vi "Vision Processing.vi"(4 "error in (no error)":errorcluster, 7 "Image Size":T1=enum."320x240") -> ()   [LabVIEW 2020]
doc: "This VI runs in parallel to other tasks. It gets images from the camera, processes them for color or shape and uses commands or globals to affect the behavior of other subsystems."
uses:
  <vilib>/Rock Robotics/WPI/Camera/WPI_CameraImageSize.ctl
  <vilib>/Rock Robotics/WPI/Camera/WPI_CameraWhite Balance Values.ctl
  <vilib>/Rock Robotics/WPI/Camera/WPI_CameraExposure Values.ctl
  <vilib>/Rock Robotics/WPI/Camera/WPI_CameraFrameRate.ctl
  Framework/Robot Global Data.vi
  <vilib>/Rock Robotics/Network Tables/NT Read Number.vi
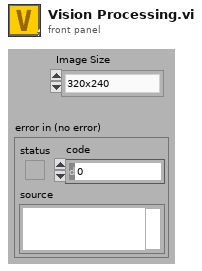
[diagram p1: front panel]
types:
  T1 = typedef "WPI_CameraImageSize.ctl" = enum16{"640x480", "320x240", "160x120", "Custom"}
  T2 = typedef "WPI_CameraFrameRate.ctl" = u32
  T3 = typedef "WPI_CameraExposure Values.ctl" = enum16{"Auto", "Flicker-free 50 Hz", "Flicker-free 60 Hz", "Hold current", "Custom"}
  T4 = typedef "WPI_CameraWhite Balance Values.ctl" = enum16{"Auto", "Fixed indoor", "Fixed outdoor 1", "Fixed outdoor 2", "Fixed fluorescent 1", "Fixed fluorescent 2", "Hold current", "Custom"}
  T5 = typedef "Image Type" = u32
  T6 = typedef "WPI_CameraDevRef.ctl" = cluster{"Camera Address":string, "CameraStatus":errorcluster}
  T7 = typedef "IMAQ Image.ctl" = refnum<image>
  T8 = typedef "WPI_ServoDeviceRef.ctl" = cluster{"DeviceStatus":errorcluster, "PWM Channel":T9, "DeadBand":T10}
  T9 = typedef "FPGA_DIOPWMChannel.ctl" = enum8{"PWM 0", "PWM 1", "PWM 2", "PWM 3", "PWM 4", "PWM 5", "PWM 6", "PWM 7", "PWM 8", "PWM 9", "PWM MXP 0", "PWM MXP 1", "PWM MXP 2", "PWM MXP 3", "PWM MXP 4", "PWM MXP 5", "PWM MXP 6", "PWM MXP 7", "PWM MXP 8", "PWM MXP 9", "Invalid"}
  T10 = typedef "WPI_PWMDeadband.ctl" = cluster{"Name":string, "maxPositivePwm":i32, "minPositivePwm":i32, "centerPwm":i32, "maxNegativePwm":i32, "minNegativePwm":i32, "angularRange":u16}
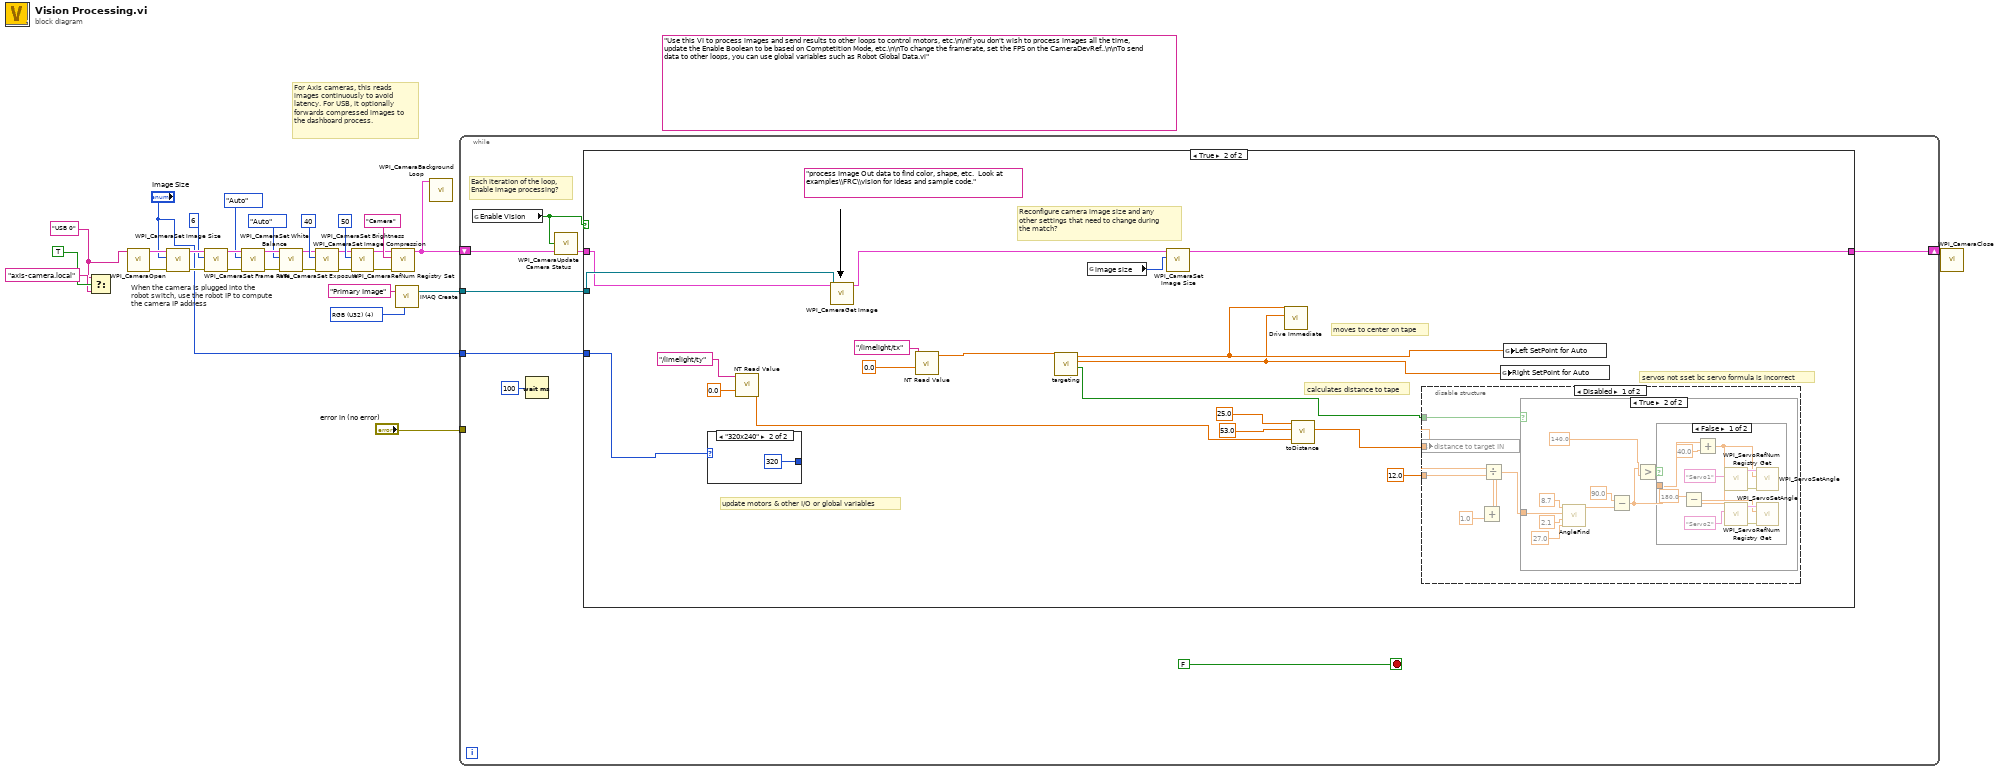
[diagram p0: block diagram]
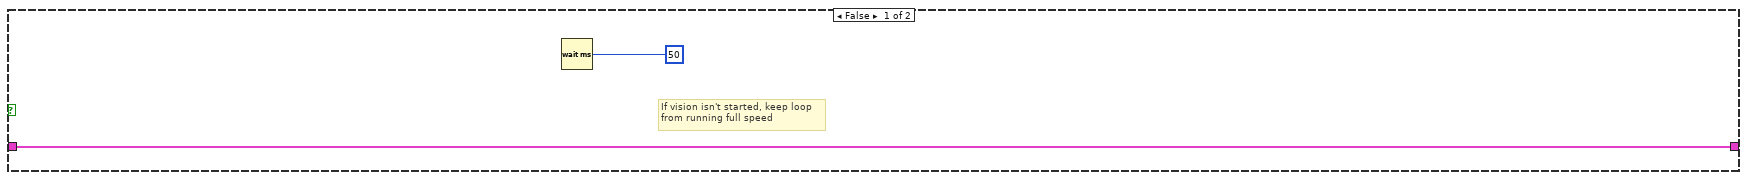
[diagram p2: hidden frame]
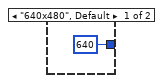
[diagram p6: hidden frame]
diagram:
  w2 = "USB 0" ("format string")
  (unwired) "Use this VI to process images and send results to other loops to control motors, etc.\n\nIf you don't wish to process images all the time, update the Enable Boolean to be based on Comptetition Mode, etc.\n\nTo change the framerate, set the FPS on the CameraDevRef..\n\nTo send data to other loops, you can use global variables such as Robot Global Data.vi"
  w30 = T5 4 items=["Grayscale (U8)", "Grayscale (I16)", "Grayscale (SGL)", "Complex (CSG)", "RGB (U32)", "HSL (U32)", "RGB (U64)"] ("Image Type")
  # "When the camera is plugged into the\nrobot switch, use the robot IP to compute\nthe camera IP address"
  # "For Axis cameras, this reads\nimages continuously to avoid\nlatency. For USB, it optionally\nforwards compressed images to\nthe dashboard process."
  n1 = Select(t=w2, s=TRUE ("dot notation? (F)"), f="axis-camera.local" ("format string")) -> ()  [unwired: 1 out]
  n2 = call <vilib>:"WPI_CameraOpen.vi"("Camera Address"=w2) -> ("error out"=w18:errorcluster, "CameraDevRef"=w19:T6)  [unwired: 2 in, 7 out]
  n3 = call <vilib>:"WPI_CameraSet Image Size.vi"("error in (no error)"=w18, "Image Size"="Image Size", "CameraDevRef"=w19) -> ("error out"=w17:errorcluster, "CameraDevRef Out"=w20:T6)  [unwired: 1 in, 6 out]
  n4 = call <vilib>:"WPI_CameraSet Frame Rate.vi"("error in (no error)"=w17, "Frame Rate (fps)"=T2 6, "CameraDevRef"=w20) -> ("error out"=w16:errorcluster, "CameraDevRef Out"=w22:T6)  [unwired: 7 out]
  n5 = call <vilib>:"WPI_CameraSet White Balance.vi"("error in (no error)"=w16, "White Balance"=WPI_CameraWhite_Balance_Values."Auto", "CameraDevRef"=w22) -> ("error out"=w15:errorcluster, "CameraDevRef Out"=w21:T6)  [unwired: 1 in, 6 out]
  n6 = call <vilib>:"WPI_CameraSet Exposure.vi"("error in (no error)"=w15, "Exposure"=WPI_CameraExposure_Values."Auto", "CameraDevRef"=w21) -> ("error out"=w14:errorcluster, "CameraDevRef Out"=w24:T6)  [unwired: 1 in, 6 out]
  n7 = call <vilib>:"WPI_CameraSet Image Compression.vi"("error in (no error)"=w14, "Compression"=40, "CameraDevRef"=w24) -> ("error out"=w13:errorcluster, "CameraDevRef Out"=w23:T6)  [unwired: 7 out]
  n8 = call <vilib>:"WPI_CameraSet Brightness.vi"("error in (no error)"=w13, "Brightness"=50, "CameraDevRef"=w23) -> ("error out"=w11:errorcluster, "CameraDevRef Out"=w12:T6)  [unwired: 1 in, 6 out]
  n9 = call <vilib>:"WPI_CameraRefNum Registry Set.vi"("error in (no error)"=w11, "refnum name"="Camera", "CameraDevRef"=w12) -> ("CameraDevRef"=w7:T6)  [unwired: 1 in, 7 out]
  n10 = call "IMAQ Create"("Image Name"="Primary Image", "Image Type"=w30) -> ("New Image"=w28:T7)  [unwired: 2 in, 2 out]
  n11 = call <vilib>:"WPI_CameraBackground Loop.vi"("CameraDevRef"=w7) -> ()  [unwired: 11 in]
  n12 = while {
    shift-right: [w37] -> w6
    shift-left: w7 -> [w35]
    tunnel: w28 -> [w36]
    tunnel: "error in (no error)" -> [_]
    tunnel: "Image Size" -> [w33]
    stop <- FALSE stop-if-true
    # "Each iteration of the loop,\nEnable image processing?"
    n13 = global read "Robot Global Data.vi" "Enable Vision"() -> (w31:bool)
    n14 = Wait (ms)(milliseconds to wait=u32 100) -> ()  [unwired: 1 out]
    n15 = call <vilib>:"WPI_CameraUpdate Camera Status.vi"("CameraDevRef In"=w35, "Enable Vision"=w31) -> ("CameraDevRef Out"=w34:T6)  [unwired: 3 in]
    n16 = case shown="True" w31 {
      tunnel: w36 -> [_ w58]
      tunnel: [w40 w59] -> w37
      tunnel: w34 -> [w40 w56]
      tunnel: w33 -> [_ w54]
      frame False {
        # "If vision isn't started, keep loop\nfrom running full speed"
        n17 = Wait (ms)(milliseconds to wait=u32 50) -> ()  [unwired: 1 out]
      }
      frame True {
        (unwired) "process Image Out data to find color, shape, etc.  Look at examples\\FRC\\vision for ideas and sample code."
        # "servos not sset bc servo formula is incorrect"
        # "moves to center on tape"
        # "calculates distance to tape"
        # "update motors & other I/O or global variables"
        # "Reconfigure camera image size and any\nother settings that need to change during\nthe match?"
        n18 = case shown="\"320x240\"" w54 {
          tunnel: [640 320] -> _
          frame "640x480", Default {
          }
          frame "320x240" {
          }
        }
        n19 = call-poly <vilib>:"NT Read Value.vi"("Default Value"=0.0, "Name"="/limelight/ty") -> ("Numeric"=w48:dbl)  [unwired: 8 in, 1 out]
        n20 = call <vilib>:"WPI_CameraGet Image.vi"("Image"=w58, "CameraDevRef"=w56) -> ("CameraDevRef Out"=w55:T6)  [unwired: 1 in, 8 out]
        n21 = call-poly <vilib>:"NT Read Value.vi"("Default Value"=0.0, "Name"="/limelight/tx") -> ("Numeric"=w51:dbl)  [unwired: 8 in, 1 out]
        n22 = call "targeting.vi"("Degreee Offset"=w51) -> ("In Range?"=w41:bool, "Right"=w44:dbl, "Left"=w45:dbl)  [unwired: 8 in]
        n23 = global read "Robot Global Data.vi" "image size"() -> (w57:T1)
        n24 = call <vilib>:"WPI_CameraSet Image Size.vi"("Image Size"=w57, "CameraDevRef"=w55) -> ("CameraDevRef Out"=w59:T6)  [unwired: 2 in, 7 out]
        n25 = call "Drive Immediate.vi"("Right Setpoint"=w44, "Left Setpoint"=w45) -> ()  [unwired: 9 in, 1 out]
        n26 = call "toDistance.vi"("height of camera off ground IN"=25.0 ("height of camera off ground"), "angle from zero camera DEGREES"=53.0 ("angle from zero camera"), "angle from fov to target IN"=w48) -> ("distance to target IN"=w43:dbl)  [unwired: 6 in]
        n27 = disable-structure shown="Disabled" {
          disable-tunnel: w41 -> [w65 _]
          disable-tunnel: w43 -> [w64 _]
          disable-tunnel: 12.0 ("y") -> [w62 _]
          frame Disabled {
            n28 = global write "Robot Global Data.vi" "distance to target IN"(w64) -> ()
            n29 = Divide(x=w64, y=w62) -> (x/y=w63:dbl)
            n30 = Add(x=w63, y=1.0) -> (x+y=w61:dbl)
            n31 = case shown="True" w65 {
              tunnel: w61 -> [_ w71]
              frame False {
              }
              frame True {
                n32 = call "AngleFind.vi"("Speed Sent (ft)"=27.0, "Distance off Ground (ft)"=2.1, "Distance to Target (Ground Distance) (ft)"=w71, "Height of Target (ft)"=8.7) -> ("Angle (Degrees?)"=w73:dbl)  [unwired: 7 in]
                n33 = Subtract(x=90.0, y=w73) -> (x-y=w66:dbl)
                n34 = Greater?(x=w66, y=140.0) -> (0:w68:bool)
                n35 = case shown="False" w68 {
                  tunnel: w66 -> [w78 _]
                  frame False {
                    n36 = Add(x=w78, y=40.0) -> (x+y=w76:dbl)
                    n37 = Subtract(x=180.0, y=w76) -> (x-y=w77:dbl)
                    n38 = call <vilib>:"WPI_ServoRefNum Registry Get.vi"("refnum name"="Servo1") -> ("error out"=w84:errorcluster, "ServoDeviceRef"=w85:T8)  [unwired: 9 in]
                    n39 = call <vilib>:"WPI_ServoRefNum Registry Get.vi"("refnum name"="Servo2") -> ("error out"=w81:errorcluster, "ServoDeviceRef"=w82:T8)  [unwired: 9 in]
                    n40 = call <vilib>:"WPI_ServoSetAngle.vi"("error in (no error)"=w84, "Angle"=w76, "ServoDeviceRef"=w85) -> ()  [unwired: 7 in, 2 out]
                    n41 = call <vilib>:"WPI_ServoSetAngle.vi"("error in (no error)"=w81, "Angle"=w77, "ServoDeviceRef"=w82) -> ()  [unwired: 7 in, 2 out]
                  }
                  frame True {
                  }
                }
              }
            }
          }
          frame Enabled {
          }
        }
        n42 = global write "Robot Global Data.vi" "Right SetPoint for Auto"(w44) -> ()
        n43 = global write "Robot Global Data.vi" "Left SetPoint for Auto"(w45) -> ()
      }
    }
  }
  n44 = call <vilib>:"WPI_CameraClose.vi"("CameraDevRef"=w6) -> ()  [unwired: 1 in, 10 out]
